vi "GetWindowTitle.vi"(8 "error in (no error)":errorcluster, 11 "WindowFrame in":refnum<class "WindowFrame.lvclass">) -> (0 "error out":errorcluster, 2 "WindowTitle":string, 3 "WindowFrame out":refnum<class "WindowFrame.lvclass">)   [LabVIEW 2021, in "WindowFrame.lvlib" / "WindowFrame.lvclass"]
uses:
  WindowFrame.lvclass
  C:/GitHub/ClassUtilities/src/ClassByRef/ClassByRef.lvclass
  ClassUtilities/src/ClassByRef/ClassByRef.lvclass/ClassByRef.ctl
  WindowFrame.lvclass/WindowFrame.ctl
  c97f9d59-0e4a-4e9d-bc5a-9aa3aa8f301a.vi
  ClassUtilities/src/ClassByRef/GetRef.vi
  Action.ctl
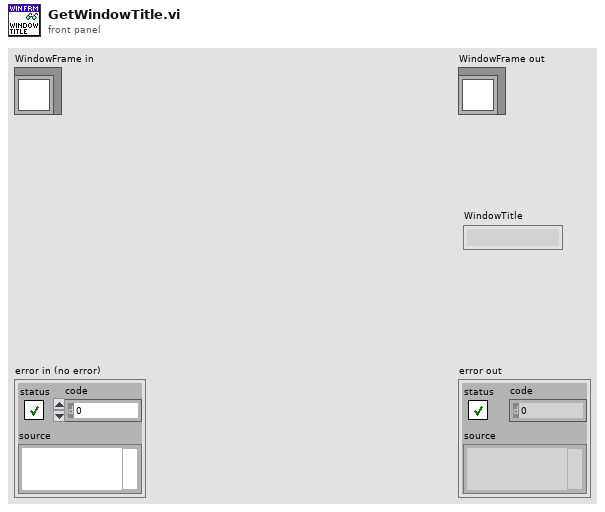
[diagram p1: front panel]
types:
  T1 = typedef "WindowFrame.lvlib/WindowFrame.lvclass/Action.ctl" = enum16{"Set Allow Runtime PopUp", "Set Behavior", "Set Closable", "Set Custom Title", "Set Highlight Return Button", "Set Is Frontmost", "Set Minimizable", "Set Minimum Size", "Set Monitor", "Set Resizable", "Set Panel Bounds", "Set Run VI Transparently", "Set Show Menu Bar", "Set State", "Set Title", "Set Title Bar Colors", "Set Title Bar Visible", "Set Transparancy", "Set Window Bounds", "Get Allow Runtime PopUp", "Get Behavior", "Get Closable", "Get Custom Title", "Get Highlight Return Button", "Get Is Frontmost", "Get Minimizable", "Get Minimum Size", "Get Monitor", "Get Panel Bounds", "Get Resizable", "Get Run VI Transparently", "Get Show Menu Bar", "Get State", "Get Title", "Get Title Bar Colors", "Get Title Bar Visible", "Get Transparancy", "Get Window Bounds", "--", "Center", "Close", "Open", "Run-Time Position:Centered", "Run-Time Position:Custom", "Run-Time Position:Get Position", "Run-Time Position:Maximized", "Run-Time Position:Minimized", "Run-Time Position:Unchanged", "---", "Insert VI", "Remove VI", "Insert VI Index", "Remove VI Index", "Exit"}
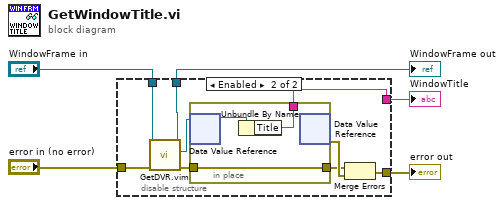
[diagram p0: block diagram]
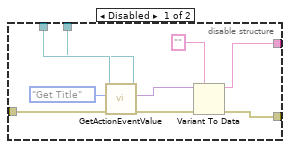
[diagram p2: hidden frame]
diagram:
  n1 = disable-structure shown="Enabled" {
    disable-tunnel: [w10 w19] -> w1
    disable-tunnel: [w9 w18] -> w4
    disable-tunnel: "error in (no error)" -> [w8 w23]
    disable-tunnel: "WindowFrame in" -> [w7 w21]
    disable-tunnel: [w6 w22] -> w2
    frame Disabled {
      n2 = call "GetActionEventValue.vi"("error in (no error)"=w8, "Action"=Action."Get Title", "WindowFrame in"=w7) -> ("error out"=w13:errorcluster, "Variant"=w12:variant, "WindowFrame out"=w6:refnum<class "WindowFrame.lvclass">)  [unwired: 6 in]
      n3 = Variant To Data(error in=w13, type="" ("Allow Runtime PopUp"), Variant=w12) -> (data=w10:string, error out=w9:errorcluster)
    }
    frame Enabled {
      n4 = call "GetDVR.vim"("error in (no error)"=w23, "ByRefClass in"=w21) -> ("error out"=w16:errorcluster, "DVR"=w20:refnum<data-value>, "ByRefClass out"=w22:refnum<class "WindowFrame.lvclass">)  [unwired: 7 in]
      n5 = in-place {
        in-place-border: [w25] -> w19
        in-place-border: [w24] -> w15
        in-place-border: w16 -> [w24]
        n6 = in-place-dvr #1(w20) -> (w26:refnum<class "WindowFrame.lvclass">)  [unwired: 1 out]
        n7 = Unbundle By Name(w26) -> ("Title"=w25:string)
        n8 = in-place-dvr #1() -> (w17:errorcluster)  [unwired: 1 in, 1 out]
      }
      n9 = Merge Errors(w15, w17) -> (w18:errorcluster)
    }
  }
  "error out" <- w4
  "WindowFrame out" <- w2
  "WindowTitle" <- w1
